vi "token_request.vi"(8 "buffer":string, 9 "url_input":string) -> (0 "body_output":string, 1 "header_output":string, 3 "client handle out":T1)   [LabVIEW 2020]
uses:
  <vilib>/httpClient/ClientHandle.ctl
  <vilib>/httpClient/POSTBuffer.vi
  <vilib>/httpClient/LabVIEWHTTPClient.lvlib
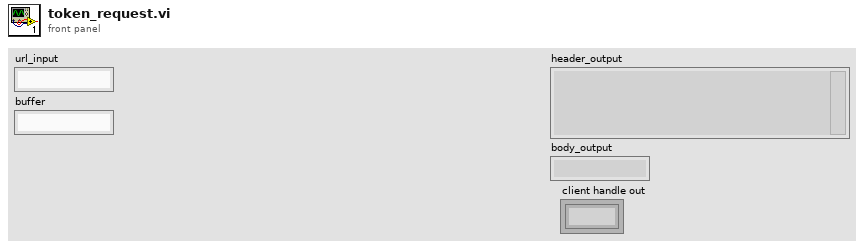
[diagram p1: front panel]
types:
  T1 = typedef "LabVIEWHTTPClient.lvlib/ClientHandle.ctl" = refnum<k1>
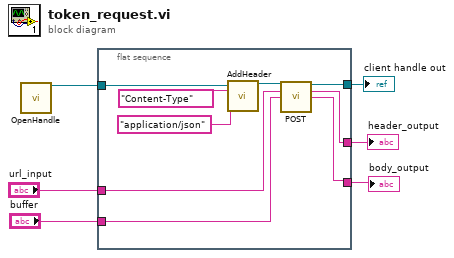
[diagram p0: block diagram]
diagram:
  n1 = call <vilib>:"OpenHandle.vi"() -> ("client handle out"=w6:T1)  [unwired: 14 in, 1 out]
  n2 = flat-sequence {
    tunnel: w6 -> [w15]
    tunnel: "buffer" -> [w11]
    tunnel: "url_input" -> [w12]
    tunnel: [w10] -> w3
    tunnel: [w8] -> w1
    tunnel: [w7] -> w2
    frame #0 {
      n3 = call <vilib>:"AddHeader.vi"("client handle"=w15, "header"="Content-Type", "value"="application/json") -> ("client handle out"=w9:T1)  [unwired: 11 in, 1 out]
      n4 = call-poly <vilib>:"POST.vi"("client handle"=w9, "url"=w12, "buffer"=w11) -> ("client handle out"=w8:T1, "headers"=w10:string, "body"=w7:string)  [unwired: 9 in, 1 out]
    }
  }
  "header_output" <- w3
  "body_output" <- w2
  "client handle out" <- w1
